vi "degree conversion-eyecursor.vi"(4 "xdegcorr":sgl, 5 "Change pupil size?":bool, 6 "1D or 2D cal?":bool, 7 "Y manual offset (degrees)":dbl, 8 "calib para":T1, 9 "pixel input":dbl[](array[numeric]), 10 "conversion factor(mm/pixel)":cluster{"x":dbl, "y":dbl}) -> (2 "angle output":dbl[](array[numeric]))   [LabVIEW 2013]
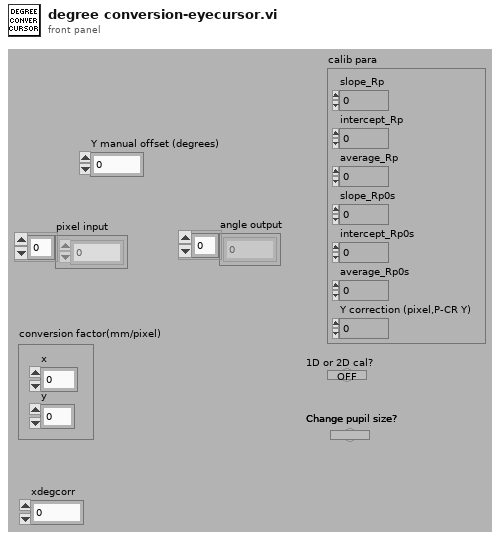
[diagram p1: front panel]
types:
  T1 = cluster{"slope_Rp":dbl, "intercept_Rp":dbl, "average_Rp":dbl, "slope_Rp0s":dbl, "intercept_Rp0s":dbl, "average_Rp0s":dbl, "Y correction (pixel,P-CR Y)":dbl}
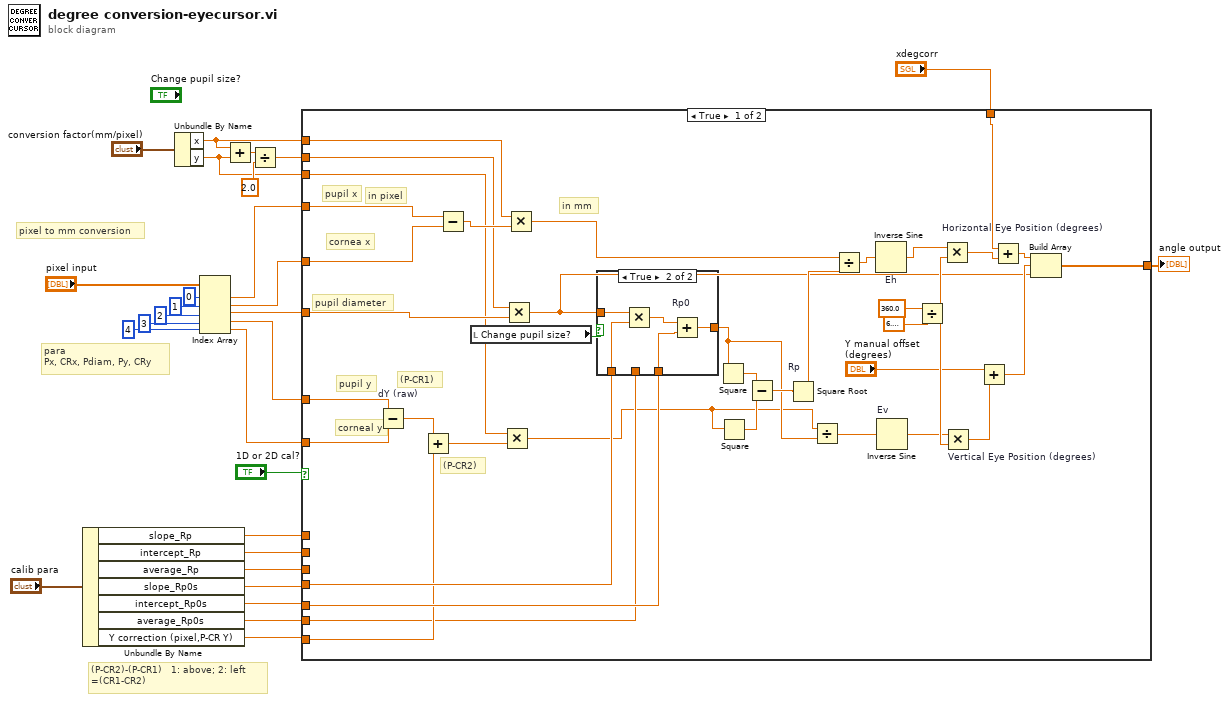
[diagram p0: block diagram]
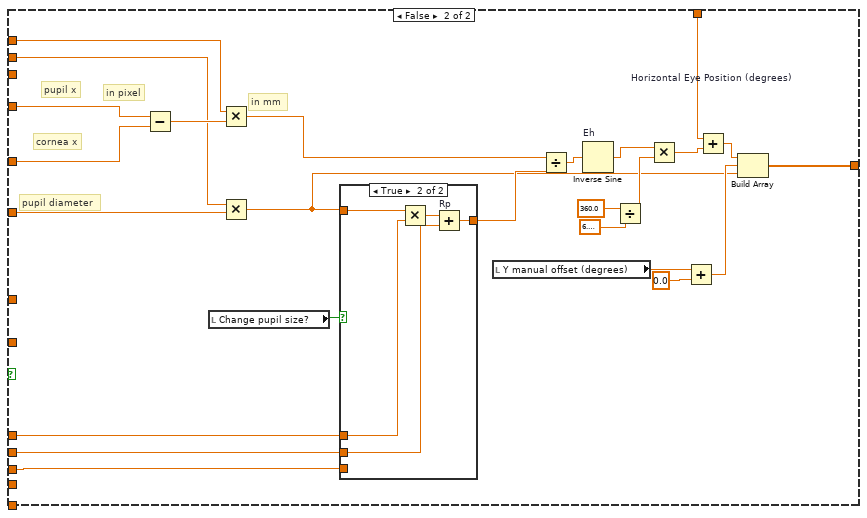
[diagram p3: hidden frame]
diagram:
  # "(P-CR2)-(P-CR1)   1: above; 2: left\n=(CR1-CR2)"
  # "para\nPx, CRx, Pdiam, Py, CRy"
  # "pixel to mm conversion"
  n1 = Unbundle By Name("calib para") -> ("slope_Rp"=w9:dbl, "intercept_Rp"=w8:dbl, "average_Rp"=w7:dbl, "slope_Rp0s"=w12:dbl, "intercept_Rp0s"=w11:dbl, "average_Rp0s"=w6:dbl, "Y correction (pixel,P-CR Y)"=w10:dbl)
  n2 = Unbundle By Name("conversion factor(mm/pixel)") -> ("x"=w4:dbl, "y"=w2:dbl)
  n3 = Index Array(array="pixel input", index #1=0 ("index"), index #2=1 ("index"), index #3=2 ("index"), index #4=3 ("index"), index #5=4 ("index")) -> (element #1=w19:dbl, element #2=w18:dbl, element #3=w17:dbl, element #4=w16:dbl, element #5=w15:dbl)
  n4 = Add(x=w4, y=w2) -> (x+y=w26:dbl)
  n5 = Divide(x=w26, y=2.0) -> (x/y=w3:dbl)
  n6 = case shown="True" "1D or 2D cal?" {
    tunnel: [w66 w97] -> w28
    tunnel: w12 -> [w59 _]
    tunnel: w11 -> [w58 _]
    tunnel: w10 -> [w50 _]
    tunnel: w19 -> [w46 w90]
    tunnel: w18 -> [w45 w89]
    tunnel: w17 -> [w40 w79]
    tunnel: w16 -> [w44 _]
    tunnel: w15 -> [w43 _]
    tunnel: w9 -> [_ w88]
    tunnel: w8 -> [_ w87]
    tunnel: w7 -> [_ w83]
    tunnel: w6 -> [w42 _]
    tunnel: w4 -> [w35 w80]
    tunnel: w3 -> [w34 w78]
    tunnel: w2 -> [w33 _]
    tunnel: "xdegcorr" -> [w29 w73]
    frame True {
      # "(P-CR2)"
      # "(P-CR1)"
      # "in mm"
      # "in pixel"
      # "corneal y"
      # "pupil y"
      # "pupil diameter"
      # "cornea x"
      # "pupil x"
      n7 = Subtract "dY (raw)"(x=w44, y=w43) -> (x-y=w57:dbl)
      n8 = Add(x=w57, y=w50) -> (x+y=w37:dbl)
      n9 = Subtract(x=w46, y=w45) -> (x-y=w39:dbl)
      n10 = local read "Change pupil size?"() -> (w41:bool)
      n11 = Multiply(x=w33, y=w37) -> (x*y=w36:dbl)
      n12 = Multiply(x=w34, y=w40) -> (x*y=w32:dbl)
      n13 = Multiply(x=w35, y=w39) -> (x*y=w38:dbl)
      n14 = case shown="True" w41 {
        tunnel: w59 -> [_ w71]
        tunnel: w58 -> [_ w70]
        tunnel: [w67 w69] -> w51
        tunnel: w32 -> [_ w68]
        tunnel: w42 -> [w67 _]
        frame False {
          # "Rp0"
        }
        frame True {
          n15 = Multiply(x=w68, y=w71) -> (x*y=w72:dbl)
          n16 = Add "Rp0"(x=w72, y=w70) -> (x+y=w69:dbl)
        }
      }
      n17 = Square(x=w51) -> (x^2=w55:dbl)
      n18 = Square(x=w36) -> (x^2=w54:dbl)
      n19 = Subtract(x=w55, y=w54) -> (x-y=w53:dbl)
      n20 = Square Root "Rp"(x=w53) -> (sqrt(x)=w52:dbl)
      n21 = Divide(x=w36, y=w51) -> (x/y=w61:dbl)
      n22 = Divide(x=w38, y=w52) -> (x/y=w63:dbl)
      n23 = Inverse Sine "Eh"(1:w63) -> (0:w62:dbl)
      n24 = Inverse Sine "Ev"(1:w61) -> (0:w56:dbl)
      n25 = Divide(x=360.0, y=6.283185307179586) -> (x/y=w60:dbl)
      n26 = Multiply "Horizontal Eye Position (degrees)"(x=w62, y=w60) -> (x*y=w30:dbl)
      n27 = Multiply "Vertical Eye Position (degrees)"(x=w56, y=w60) -> (x*y=w49:dbl)
      n28 = Add(x="Y manual offset (degrees)", y=w49) -> (x+y=w47:dbl)
      n29 = Add(x=w29, y=w30) -> (x+y=w31:dbl)
      n30 = Build Array(w31, w47, w32) -> (w66:dbl[])
    }
    frame False {
      # "in mm"
      # "in pixel"
      # "pupil diameter"
      # "cornea x"
      # "pupil x"
      n31 = Subtract(x=w90, y=w89) -> (x-y=w82:dbl)
      n32 = local read "Change pupil size?"() -> (w84:bool)
      n33 = Multiply(x=w80, y=w82) -> (x*y=w81:dbl)
      n34 = Multiply(x=w78, y=w79) -> (x*y=w76:dbl)
      n35 = case shown="True" w84 {
        tunnel: w76 -> [_ w102]
        tunnel: w88 -> [_ w101]
        tunnel: w87 -> [_ w100]
        tunnel: [w98 w99] -> w86
        tunnel: w83 -> [w98 _]
        frame False {
        }
        frame True {
          n36 = Multiply(x=w102, y=w101) -> (x*y=w103:dbl)
          n37 = Add "Rp"(x=w103, y=w100) -> (x+y=w99:dbl)
        }
      }
      n38 = local read "Y manual offset (degrees)"() -> (w85:dbl)
      n39 = Divide(x=w81, y=w86) -> (x/y=w94:dbl)
      n40 = Inverse Sine "Eh"(1:w94) -> (0:w93:dbl)
      n41 = Divide(x=360.0, y=6.283185307179586) -> (x/y=w92:dbl)
      n42 = Multiply "Horizontal Eye Position (degrees)"(x=w93, y=w92) -> (x*y=w75:dbl)
      n43 = Add(x=w85, y=0.0 ("x")) -> (x+y=w91:dbl)
      n44 = Add(x=w73, y=w75) -> (x+y=w74:dbl)
      n45 = Build Array(w74, w91, w76) -> (w97:dbl[])
    }
  }
  "angle output" <- w28
